vi "PH_Img_BaseClass.ProcPeriodic.vi"(0 "i ref in":refnum<vi>, 3 "ms timeout (10000)":i32=10000, 5 "error in (no error)":errorcluster) -> (14 "i ref out":refnum<vi>, 16 "Cam Image":T1, 17 "timed out?":bool, 18 "Error while unflatten data?":bool, 19 "error out":errorcluster)   [LabVIEW 2014, in "PH_Img_BaseClass.lvlib"]
doc: "This method serves to periodically do things like reading values from the HW. Methods that should be executed periodically should be called from THIS methode. Add code here."
uses:
  PH_Img_BaseClass.lvlib
  <vilib>/vision/Image Controls.llb/IMAQ Image.ctl
  PH_Common/PH_Common.lvlib
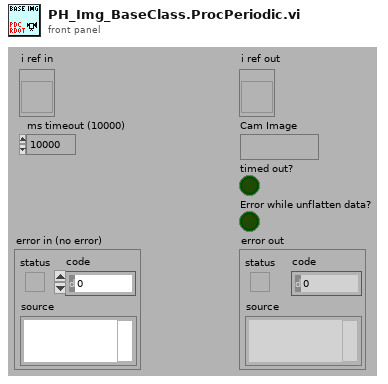
[diagram p1: front panel]
types:
  T1 = typedef "IMAQ Image.ctl" = refnum<image>
  T2 = typedef "PH_Img_BaseClass.lvlib/PH_Img_BaseClass.i attribute.ctl" = cluster{"GUI Refs":T3, "Timeout Image [ms]":i32, "Default Periodic Period [ms]":i32, "Camera":cluster{"Instancename":string, "Notifier":refnum<notifier>}, "Palette":T4, "Cam Settings":cluster{"Cam ID":string, "Gain":dbl, "Brightness":dbl, "Shutter":dbl, "Cam Info Failure":bool, "Mode":i32}}
  T3 = typedef "PH_Img_BaseClass.lvlib/PH_Img_BaseClass.GUI Refs.ctl" = cluster{"Timeout":refnum<vi>, "Image":refnum<vi>, "Palette":refnum<vi>, "Timeout Set":refnum<vi>}
  T4 = typedef "PH_Img_BaseClass.lvlib/PH_Img_BaseClass.Palette.ctl" = i32
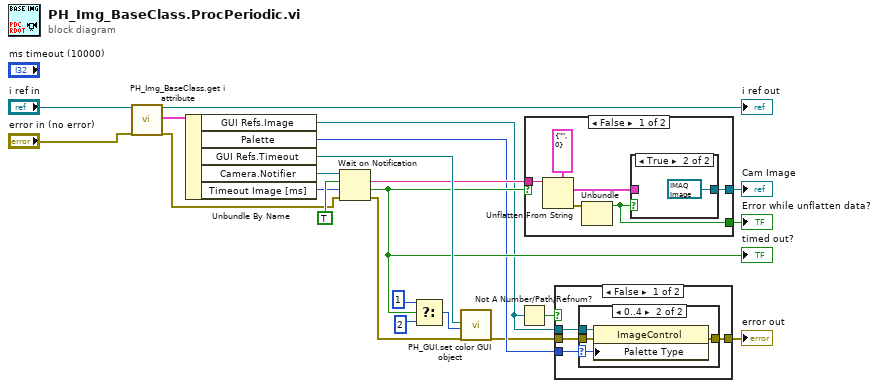
[diagram p0: block diagram]
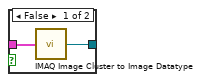
[diagram p4: hidden frame]
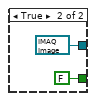
[diagram p5: hidden frame]
diagram:
  n1 = call "PH_Img_BaseClass.get i attribute.vi"("i ref in"="i ref in", "error in (no error)"="error in (no error)") -> ("i ref out"=→"i ref out":refnum<vi>, "i attribute"=w22:T2, "error out"=w17:errorcluster)  [unwired: 15 in]
  n2 = Unbundle By Name(w22) -> ("GUI Refs.Image"=w1:refnum<vi>, "Palette"=w5:T4, "GUI Refs.Timeout"=w19:refnum<vi>, "Camera.Notifier"=w18:refnum<notifier>, "Timeout Image [ms]"=w20:i32)
  n3 = Wait on Notification(notifier=w18, ignore previous (F)=TRUE, timeout in ms (-1)=w20, error in (no error)=w17) -> (notification=w9:string, timed out?=w6:bool, error out=w10:errorcluster)  [unwired: 1 out]
  "timed out?" <- w6
  n4 = Select(t=1, s=w6, f=2) -> (s? t:f=w12:i32)
  n5 = call "PH_GUI.set color GUI object.vi"("GUI object Ref"=w19, "State"=w12, "error in (no error)"=w10) -> ("error out"=w4:errorcluster)  [unwired: 16 in]
  n6 = Not A Number/Path/Refnum?(number/path/refnum=w1) -> (NaN/Path/Refnum?=w2:bool)
  n7 = case shown="False" w6 {
    tunnel: w9 -> [w25 _]
    tunnel: [w23 FALSE ("status")] -> w8
    tunnel: [w24 T1 refnum ("Image (dup)")] -> w7
    frame False {
      n8 = Unflatten From String(type=cluster{string, u32} {"", 0} ("Image Out"), binary string=w25) -> (value=w26:cluster{string, u32}, error out=w27:errorcluster)  [unwired: 3 in, 1 out]
      n9 = Unbundle(w27) -> ("status"=w23:bool)  [unwired: 2 out]
      n10 = case shown="True" w23 {
        tunnel: w26 -> [w30 _]
        tunnel: [w29 T1 refnum ("Image (dup)")] -> w24
        frame False {
          n11 = call <vilib>:"IMAQ Image Cluster to Image Datatype.vi"("Image"=w30) -> ("Image (dup)"=w29:T1)
        }
        frame True {
        }
      }
    }
    frame True {
    }
  }
  "Cam Image" <- w7
  "Error while unflatten data?" <- w8
  n12 = case shown="False" w2 {
    tunnel: w1 -> [w37 _]
    tunnel: w5 -> [w36 _]
    tunnel: [w35 w43] -> w3
    tunnel: w4 -> [w34 w43]
    frame False {
      n13 = case shown="0..4" w36 {
        selector: w36 -> [_ w41]
        tunnel: w37 -> [_ w42]
        tunnel: [w38 w40] -> w35
        tunnel: w34 -> [w38 w39]
        frame Default {
        }
        frame 0..4 {
          n14 = property class="ImageControl"(reference=w42, error in=w39, "Palette Type"=w41) -> (error out=w40:errorcluster)  [unwired: 1 out]
        }
      }
    }
    frame True {
    }
  }
  "error out" <- w3
